vi "LSMcontroller_v59_PIzstage.vi"() -> ()   [LabVIEW 2015] (continued)
                        n916 = local write "64bit disabled"(TRUE ("64bit disabled")) -> ()
                      }
                      frame #9 {
                        n917 = call "2pparameters.vi"("command"="get") -> ("params out"=w3214:T11)  [unwired: 1 in]
                        n918 = Unbundle By Name(w3214) -> ("auto OD"=w3213:bool)
                        n919 = case shown="True" w3213 {
                          frame False {
                          }
                          frame True {
                            n920 = call "configuration.vi"("command"="get") -> ("config out"=w3217:T12)  [unwired: 2 in, 1 out]
                            n921 = call "2pparameters.vi"("command"="get") -> ("params out"=w3220:T11)  [unwired: 1 in]
                            n922 = Unbundle By Name(w3217) -> ("image OD"=w3215:u16)
                            n923 = Unbundle By Name(w3220) -> ("ODfilt"=w3216:u16)
                            n924 = call "filterwheelcontrol_nothorlabslib.vi"("Current OD filt"=w3215, "New ODfilt"=w3216) -> ()  [unwired: 1 in]
                          }
                        }
                        n925 = call "reset AO_DO_v3.vi"() -> ()  [unwired: 12 in]
                      }
                      frame #10 {
                        n926 = stacked-sequence {
                          tunnel: w3234 -> [w3237 _ _ _ _ _]
                          tunnel: w3233 -> [w3236 _ _ _ _ _]
                          tunnel: w3232 -> [w3235 _ _ _ _ _]
                          tunnel: w3231 -> [_ w3286 _ _ _ _]
                          tunnel: w3230 -> [_ w3285 w3340 w3437 _ _]
                          tunnel: w3229 -> [_ w3284 w3339 w3436 _ _]
                          tunnel: w3228 -> [_ _ w3338 _ _ _]
                          tunnel: w3227 -> [_ _ w3337 _ _ _]
                          tunnel: w3226 -> [_ _ _ w3435 _ _]
                          tunnel: w3225 -> [_ _ _ w3434 _ _]
                          tunnel: w3224 -> [_ _ w3335 _ _ _]
                          tunnel: w3223 -> [_ _ w3334 _ _ _]
                          tunnel: w3222 -> [_ _ _ w3432 _ _]
                          tunnel: w3221 -> [_ _ _ w3431 _ _]
                          frame #0 {
                            n927 = case shown="False" w3237 {
                              tunnel: w3236 -> [_ w3259]
                              tunnel: w3235 -> [_ w3258]
                              frame True {
                                n928 = stacked-sequence {
                                seq-local: [w3238 _ _] -> [_ w3250 w3255]
                                frame #0 {
                                n929 = call "configuration.vi"("command"="get") -> ("config out"=w3244:T12)  [unwired: 2 in, 1 out]
                                n930 = Unbundle By Name(w3244) -> ("Voltage to Xgalvo"=w3241:i32)
                                n931 = call "2pparameters.vi"("command"="get") -> ("params out"=w3242:T11)  [unwired: 1 in]
                                n932 = in-place {
                                in-place-border: w3241 -> [w3249]
                                in-place-border: [w3246] -> w3238
                                n933 = in-place-cluster #9(w3242) -> ("aAO"=w3248:u32[])
                                n934 = call "remove channel from active arrayv2.vi"("line array in"=w3248, "line to remove"=w3249) -> ("line array out"=w3247:u32[], "index"=w3246:i32)  [unwired: 1 out]
                                n935 = in-place-cluster #9("aAO"=w3247) -> (w3239:T11)
                                }
                                n936 = call "2pparameters.vi"("Params in"=w3239, "command"="set") -> ()  [unwired: 1 out]
                                }
                                frame #1 {
                                n937 = call "waveformparamsv2.vi"("command"="rem AO", "index"=w3250) -> ()  [unwired: 3 in, 3 out]
                                }
                                frame #2 {
                                n938 = call "waveformsAObuffer.vi"("command"="get") -> ("AO wf out"=w3256:waveform(dbl)[])  [unwired: 1 in]
                                n939 = Delete From Array(array=w3256, length=1, index=w3255) -> (array with subset deleted=w3252:waveform(dbl)[])  [unwired: 1 out]
                                n940 = call "waveformsAObuffer.vi"("AO wf in"=w3252, "command"="set") -> ()  [unwired: 1 out]
                                }
                                }
                              }
                              frame False {
                                n941 = stacked-sequence {
                                seq-local: [w3260 _ _] -> [_ w3268 w3279]
                                tunnel: w3259 -> [_ w3267 _]
                                tunnel: w3258 -> [_ _ w3278]
                                frame #0 {
                                n942 = call "configuration.vi"("command"="get") -> ("config out"=w3265:T12)  [unwired: 2 in, 1 out]
                                n943 = Unbundle By Name(w3265) -> ("Voltage to Xgalvo"=w3261:i32)
                                n944 = call "2pparameters.vi"("command"="get") -> ("params out"=w3264:T11)  [unwired: 1 in]
                                n945 = Unbundle By Name(w3264) -> ("aAO"=w3262:u32[])
                                n946 = Search 1D Array(1D array=w3262, element=w3261) -> (index of element=w3260:i32)  [unwired: 1 in]
                                }
                                frame #1 {
                                n947 = call "waveformparamsv2.vi"("command"="get") -> ("Params out"=w3271:T15)  [unwired: 4 in, 2 out]
                                n948 = in-place {
                                in-place-border: w3268 -> [w3275]
                                in-place-border: w3267 -> [w3274]
                                n949 = in-place-cluster #10(w3271) -> ("AO parameters"=w3276:T16)
                                n950 = in-place {
                                in-place-border: w3274 -> [w3277]
                                n951 = in-place-array #11(w3276, w3275) -> ()  [unwired: 1 out]
                                n952 = in-place-array #11(w3277) -> (w3273:T16)  [unwired: 1 out]
                                }
                                n953 = in-place-cluster #10("AO parameters"=w3273) -> (w3269:T15)
                                }
                                n954 = call "waveformparamsv2.vi"("command"="set", "Params in"=w3269) -> ()  [unwired: 3 in, 3 out]
                                }
                                frame #2 {
                                n955 = call "waveformsAObuffer.vi"("command"="get") -> ("AO wf out"=w3282:waveform(dbl)[])  [unwired: 1 in]
                                n956 = Replace Array Subset(array=w3282, new element=w3278, index=w3279) -> (w3280:waveform(dbl)[])
                                n957 = call "waveformsAObuffer.vi"("AO wf in"=w3280, "command"="set") -> ()  [unwired: 1 out]
                                }
                                }
                              }
                            }
                          }
                          frame #1 {
                            n958 = case shown="True" w3286 {
                              tunnel: w3285 -> [_ w3308]
                              tunnel: w3284 -> [_ w3307]
                              frame True {
                                n959 = stacked-sequence {
                                seq-local: [w3287 _ _] -> [_ w3299 w3304]
                                frame #0 {
                                n960 = call "configuration.vi"("command"="get") -> ("config out"=w3293:T12)  [unwired: 2 in, 1 out]
                                n961 = Unbundle By Name(w3293) -> ("Voltage to Ygalvo"=w3290:i32)
                                n962 = call "2pparameters.vi"("command"="get") -> ("params out"=w3291:T11)  [unwired: 1 in]
                                n963 = in-place {
                                in-place-border: w3290 -> [w3298]
                                in-place-border: [w3295] -> w3287
                                n964 = in-place-cluster #12(w3291) -> ("aAO"=w3297:u32[])
                                n965 = call "remove channel from active arrayv2.vi"("line array in"=w3297, "line to remove"=w3298) -> ("line array out"=w3296:u32[], "index"=w3295:i32)  [unwired: 1 out]
                                n966 = in-place-cluster #12("aAO"=w3296) -> (w3288:T11)
                                }
                                n967 = call "2pparameters.vi"("Params in"=w3288, "command"="set") -> ()  [unwired: 1 out]
                                }
                                frame #1 {
                                n968 = call "waveformparamsv2.vi"("command"="rem AO", "index"=w3299) -> ()  [unwired: 3 in, 3 out]
                                }
                                frame #2 {
                                n969 = call "waveformsAObuffer.vi"("command"="get") -> ("AO wf out"=w3305:waveform(dbl)[])  [unwired: 1 in]
                                n970 = Delete From Array(array=w3305, length=1, index=w3304) -> (array with subset deleted=w3301:waveform(dbl)[])  [unwired: 1 out]
                                n971 = call "waveformsAObuffer.vi"("AO wf in"=w3301, "command"="set") -> ()  [unwired: 1 out]
                                }
                                }
                              }
                              frame False {
                                n972 = stacked-sequence {
                                seq-local: [w3309 _ _] -> [_ w3317 w3328]
                                tunnel: w3308 -> [_ w3316 _]
                                tunnel: w3307 -> [_ _ w3327]
                                frame #0 {
                                n973 = call "configuration.vi"("command"="get") -> ("config out"=w3314:T12)  [unwired: 2 in, 1 out]
                                n974 = Unbundle By Name(w3314) -> ("Voltage to Ygalvo"=w3310:i32)
                                n975 = call "2pparameters.vi"("command"="get") -> ("params out"=w3313:T11)  [unwired: 1 in]
                                n976 = Unbundle By Name(w3313) -> ("aAO"=w3311:u32[])
                                n977 = Search 1D Array(1D array=w3311, element=w3310) -> (index of element=w3309:i32)  [unwired: 1 in]
                                }
                                frame #1 {
                                n978 = call "waveformparamsv2.vi"("command"="get") -> ("Params out"=w3320:T15)  [unwired: 4 in, 2 out]
                                n979 = in-place {
                                in-place-border: w3317 -> [w3324]
                                in-place-border: w3316 -> [w3323]
                                n980 = in-place-cluster #13(w3320) -> ("AO parameters"=w3325:T16)
                                n981 = in-place {
                                in-place-border: w3323 -> [w3326]
                                n982 = in-place-array #14(w3325, w3324) -> ()  [unwired: 1 out]
                                n983 = in-place-array #14(w3326) -> (w3322:T16)  [unwired: 1 out]
                                }
                                n984 = in-place-cluster #13("AO parameters"=w3322) -> (w3318:T15)
                                }
                                n985 = call "waveformparamsv2.vi"("command"="set", "Params in"=w3318) -> ()  [unwired: 3 in, 3 out]
                                }
                                frame #2 {
                                n986 = call "waveformsAObuffer.vi"("command"="get") -> ("AO wf out"=w3331:waveform(dbl)[])  [unwired: 1 in]
                                n987 = Replace Array Subset(array=w3331, new element=w3327, index=w3328) -> (w3329:waveform(dbl)[])
                                n988 = call "waveformsAObuffer.vi"("AO wf in"=w3329, "command"="set") -> ()  [unwired: 1 out]
                                }
                                }
                              }
                            }
                          }
                          frame #2 {
                            n989 = Build Array(w3335, w3334) -> (w3333:bool[])
                            n990 = Boolean Array To Number(Boolean array=w3333) -> (number=w3336:u32)
                            n991 = case shown="0" w3336 {
                              tunnel: w3340 -> [_ _ w3383]
                              tunnel: w3339 -> [_ _ w3382]
                              tunnel: w3338 -> [_ w3362 w3380]
                              tunnel: w3337 -> [_ w3361 w3381]
                              frame 1, Default {
                                n992 = stacked-sequence {
                                seq-local: [w3341 _ _] -> [_ w3353 w3358]
                                frame #0 {
                                n993 = call "configuration.vi"("command"="get") -> ("config out"=w3347:T12)  [unwired: 2 in, 1 out]
                                n994 = Unbundle By Name(w3347) -> ("2P shutter"=w3344:i32)
                                n995 = call "2pparameters.vi"("command"="get") -> ("params out"=w3345:T11)  [unwired: 1 in]
                                n996 = in-place {
                                in-place-border: w3344 -> [w3352]
                                in-place-border: [w3349] -> w3341
                                n997 = in-place-cluster #15(w3345) -> ("aDO"=w3351:u32[])
                                n998 = call "remove channel from active arrayv2.vi"("line array in"=w3351, "line to remove"=w3352) -> ("line array out"=w3350:u32[], "index"=w3349:i32)  [unwired: 1 out]
                                n999 = in-place-cluster #15("aDO"=w3350) -> (w3342:T11)
                                }
                                n1000 = call "2pparameters.vi"("Params in"=w3342, "command"="set") -> ()  [unwired: 1 out]
                                }
                                frame #1 {
                                n1001 = call "waveformparamsv2.vi"("command"="rem DO", "index"=w3353) -> ()  [unwired: 3 in, 3 out]
                                }
                                frame #2 {
                                n1002 = call "waveformsDObuffer.vi"("command"="get") -> ("DO wf out"=w3359:digitalwaveform[])  [unwired: 1 in]
                                n1003 = Delete From Array(array=w3359, length=1, index=w3358) -> (array with subset deleted=w3355:digitalwaveform[])  [unwired: 1 out]
                                n1004 = call "waveformsDObuffer.vi"("DO wf in"=w3355, "command"="set") -> ()  [unwired: 1 out]
                                }
                                }
                              }
                              frame 2 {
                                n1005 = stacked-sequence {
                                tunnel: w3362 -> [_ w3373 _]
                                tunnel: w3361 -> [_ _ w3377]
                                frame #0 {
                                n1006 = call "configuration.vi"("command"="get") -> ("config out"=w3364:T12)  [unwired: 2 in, 1 out]
                                n1007 = call "2pparameters.vi"("command"="get") -> ("params out"=w3368:T11)  [unwired: 1 in]
                                n1008 = Unbundle By Name(w3364) -> ("2P shutter"=w3363:i32)
                                n1009 = in-place {
                                in-place-border: w3363 -> [w3372]
                                n1010 = in-place-cluster #16(w3368) -> ("aDO"=w3371:u32[])
                                n1011 = call "add channel to active arrayv2.vi"("line array in"=w3371, "line to add"=w3372) -> ("line array out"=w3370:u32[])  [unwired: 2 out]
                                n1012 = in-place-cluster #16("aDO"=w3370) -> (w3366:T11)
                                }
                                n1013 = call "2pparameters.vi"("Params in"=w3366, "command"="set") -> ()  [unwired: 1 out]
                                }
                                frame #1 {
                                n1014 = call "waveformparamsv2.vi"("command"="add DO", "add DO"=w3373) -> ()  [unwired: 3 in, 3 out]
                                }
                                frame #2 {
                                n1015 = call "waveformsDObuffer.vi"("command"="get") -> ("DO wf out"=w3378:digitalwaveform[])  [unwired: 1 in]
                                n1016 = Build Array (concatenate)(w3378, w3377) -> (w3376:digitalwaveform[])
                                n1017 = call "waveformsDObuffer.vi"("DO wf in"=w3376, "command"="set") -> ()  [unwired: 1 out]
                                }
                                }
                              }
                              frame 0 {
                                n1018 = stacked-sequence {
                                seq-local: [w3384 _ _] -> [_ w3392 w3414]
                                tunnel: w3383 -> [_ _ _]
                                tunnel: w3382 -> [_ _ _]
                                tunnel: w3381 -> [_ _ w3413]
                                tunnel: w3380 -> [_ w3391 _]
                                frame #0 {
                                n1019 = call "configuration.vi"("command"="get") -> ("config out"=w3389:T12)  [unwired: 2 in, 1 out]
                                n1020 = call "2pparameters.vi"("command"="get") -> ("params out"=w3388:T11)  [unwired: 1 in]
                                n1021 = Unbundle By Name(w3389) -> ("2P shutter"=w3385:i32)
                                n1022 = Unbundle By Name(w3388) -> ("aDO"=w3386:u32[])
                                n1023 = Search 1D Array(1D array=w3386, element=w3385) -> (index of element=w3384:i32)  [unwired: 1 in]
                                }
                                frame #1 {
                                n1024 = call "2pparameters.vi"("command"="get") -> ("params out"=w3395:T11)  [unwired: 1 in]
                                n1025 = Unbundle By Name(w3395) -> ("wavdet"=w3393:bool, "autoshutter"=w3394:bool)
                                n1026 = case shown="True" w3394 {
                                tunnel: w3392 -> [_ w3399]
                                tunnel: w3393 -> [_ w3398]
                                tunnel: w3391 -> [_ w3397]
                                frame False {
                                }
                                frame True {
                                n1027 = case shown="False" w3398 {
                                tunnel: w3399 -> [w3403 _]
                                tunnel: w3397 -> [w3401 _]
                                frame False {
                                n1028 = Index Array(array=w3401, index=0) -> (element=w3400:T19)
                                n1029 = call "waveformparamsv2.vi"("command"="get") -> ("Params out"=w3406:T15)  [unwired: 4 in, 2 out]
                                n1030 = in-place {
                                in-place-border: w3403 -> [w3410]
                                in-place-border: w3400 -> [w3408]
                                n1031 = in-place-cluster #17(w3406) -> ("DO parameters"=w3411:T18)
                                n1032 = in-place {
                                in-place-border: w3408 -> [w3412]
                                n1033 = in-place-array #18(w3411, w3410) -> ()  [unwired: 1 out]
                                n1034 = in-place-array #18(w3412) -> (w3409:T18)  [unwired: 1 out]
                                }
                                n1035 = in-place-cluster #17("DO parameters"=w3409) -> (w3404:T15)
                                }
                                n1036 = call "waveformparamsv2.vi"("command"="set", "Params in"=w3404) -> ()  [unwired: 3 in, 3 out]
                                }
                                frame True {
                                }
                                }
                                }
                                }
                                }
                                frame #2 {
                                n1037 = call "2pparameters.vi"("command"="get") -> ("params out"=w3417:T11)  [unwired: 1 in]
                                n1038 = Unbundle By Name(w3417) -> ("wavdet"=w3415:bool, "autoshutter"=w3416:bool)
                                n1039 = case shown="True" w3416 {
                                tunnel: w3414 -> [_ w3421]
                                tunnel: w3415 -> [_ w3420]
                                tunnel: w3413 -> [_ w3419]
                                frame False {
                                }
                                frame True {
                                n1040 = case shown="False" w3420 {
                                tunnel: w3421 -> [w3425 _]
                                tunnel: w3419 -> [w3424 _]
                                frame False {
                                n1041 = Index Array(array=w3424, index=0) -> (element=w3422:digitalwaveform)
                                n1042 = call "waveformsDObuffer.vi"("command"="get") -> ("DO wf out"=w3427:digitalwaveform[])  [unwired: 1 in]
                                n1043 = Replace Array Subset(array=w3427, new element=w3422, index=w3425) -> (w3429:digitalwaveform[])
                                n1044 = call "waveformsDObuffer.vi"("DO wf in"=w3429, "command"="set") -> ()  [unwired: 1 out]
                                }
                                frame True {
                                }
                                }
                                }
                                }
                                }
                                }
                              }
                            }
                          }
                          frame #3 {
                            n1045 = Build Array(w3432, w3431) -> (w3433:bool[])
                            n1046 = Boolean Array To Number(Boolean array=w3433) -> (number=w3430:u32)
                            n1047 = case shown="0" w3430 {
                              tunnel: w3437 -> [_ _ w3480]
                              tunnel: w3436 -> [_ _ w3479]
                              tunnel: w3435 -> [_ w3459 w3477]
                              tunnel: w3434 -> [_ w3458 w3478]
                              frame 1, Default {
                                n1048 = stacked-sequence {
                                seq-local: [w3438 _ _] -> [_ w3450 w3455]
                                frame #0 {
                                n1049 = call "configuration.vi"("command"="get") -> ("config out"=w3444:T12)  [unwired: 2 in, 1 out]
                                n1050 = Unbundle By Name(w3444) -> ("LT timestamp"=w3441:u32)
                                n1051 = call "2pparameters.vi"("command"="get") -> ("params out"=w3442:T11)  [unwired: 1 in]
                                n1052 = in-place {
                                in-place-border: w3441 -> [w3449]
                                in-place-border: [w3446] -> w3438
                                n1053 = in-place-cluster #19(w3442) -> ("aDO"=w3448:u32[])
                                n1054 = call "remove channel from active arrayv2.vi"("line array in"=w3448, "line to remove"=w3449) -> ("line array out"=w3447:u32[], "index"=w3446:i32)  [unwired: 1 out]
                                n1055 = in-place-cluster #19("aDO"=w3447) -> (w3439:T11)
                                }
                                n1056 = call "2pparameters.vi"("Params in"=w3439, "command"="set") -> ()  [unwired: 1 out]
                                }
                                frame #1 {
                                n1057 = call "waveformparamsv2.vi"("command"="rem DO", "index"=w3450) -> ()  [unwired: 3 in, 3 out]
                                }
                                frame #2 {
                                n1058 = call "waveformsDObuffer.vi"("command"="get") -> ("DO wf out"=w3456:digitalwaveform[])  [unwired: 1 in]
                                n1059 = Delete From Array(array=w3456, length=1, index=w3455) -> (array with subset deleted=w3452:digitalwaveform[])  [unwired: 1 out]
                                n1060 = call "waveformsDObuffer.vi"("DO wf in"=w3452, "command"="set") -> ()  [unwired: 1 out]
                                }
                                }
                              }
                              frame 2 {
                                n1061 = stacked-sequence {
                                tunnel: w3459 -> [_ _ w3472]
                                tunnel: w3458 -> [_ w3470 _]
                                frame #0 {
                                n1062 = call "configuration.vi"("command"="get") -> ("config out"=w3461:T12)  [unwired: 2 in, 1 out]
                                n1063 = Unbundle By Name(w3461) -> ("LT timestamp"=w3460:u32)
                                n1064 = call "2pparameters.vi"("command"="get") -> ("params out"=w3465:T11)  [unwired: 1 in]
                                n1065 = in-place {
                                in-place-border: w3460 -> [w3469]
                                n1066 = in-place-cluster #20(w3465) -> ("aDO"=w3468:u32[])
                                n1067 = call "add channel to active arrayv2.vi"("line array in"=w3468, "line to add"=w3469) -> ("line array out"=w3467:u32[])  [unwired: 2 out]
                                n1068 = in-place-cluster #20("aDO"=w3467) -> (w3463:T11)
                                }
                                n1069 = call "2pparameters.vi"("Params in"=w3463, "command"="set") -> ()  [unwired: 1 out]
                                }
                                frame #1 {
                                n1070 = call "waveformparamsv2.vi"("command"="add DO", "add DO"=w3470) -> ()  [unwired: 3 in, 3 out]
                                }
                                frame #2 {
                                n1071 = call "waveformsDObuffer.vi"("command"="get") -> ("DO wf out"=w3475:digitalwaveform[])  [unwired: 1 in]
                                n1072 = Build Array (concatenate)(w3475, w3472) -> (w3474:digitalwaveform[])
                                n1073 = call "waveformsDObuffer.vi"("DO wf in"=w3474, "command"="set") -> ()  [unwired: 1 out]
                                }
                                }
                              }
                              frame 0 {
                                n1074 = stacked-sequence {
                                seq-local: [w3481 _ _] -> [_ w3491 w3508]
                                tunnel: w3480 -> [_ _ _]
                                tunnel: w3479 -> [_ _ _]
                                tunnel: w3478 -> [_ w3488 _]
                                tunnel: w3477 -> [_ _ w3507]
                                frame #0 {
                                n1075 = call "configuration.vi"("command"="get") -> ("config out"=w3486:T12)  [unwired: 2 in, 1 out]
                                n1076 = Unbundle By Name(w3486) -> ("LT timestamp"=w3482:u32)
                                n1077 = call "2pparameters.vi"("command"="get") -> ("params out"=w3485:T11)  [unwired: 1 in]
                                n1078 = Unbundle By Name(w3485) -> ("aDO"=w3483:u32[])
                                n1079 = Search 1D Array(1D array=w3483, element=w3482) -> (index of element=w3481:i32)  [unwired: 1 in]
                                }
                                frame #1 {
                                n1080 = local read "Measurement"() -> (w3490:T4)
                                n1081 = To Unsigned Long Integer(number=w3490) -> (unsigned 32bit integer=w3489:u32)
                                n1082 = case shown="5..7" w3489 {
                                tunnel: w3491 -> [_ w3495]
                                tunnel: w3488 -> [_ w3492]
                                frame 0..4, Default {
                                }
                                frame 5..7 {
                                n1083 = Index Array(array=w3492, index=0) -> (element=w3493:T19)
                                n1084 = call "waveformparamsv2.vi"("command"="get") -> ("Params out"=w3498:T15)  [unwired: 4 in, 2 out]
                                n1085 = in-place {
                                in-place-border: w3495 -> [w3502]
                                in-place-border: w3493 -> [w3500]
                                n1086 = in-place-cluster #21(w3498) -> ("DO parameters"=w3503:T18)
                                n1087 = in-place {
                                in-place-border: w3500 -> [w3504]
                                n1088 = in-place-array #22(w3503, w3502) -> ()  [unwired: 1 out]
                                n1089 = in-place-array #22(w3504) -> (w3501:T18)  [unwired: 1 out]
                                }
                                n1090 = in-place-cluster #21("DO parameters"=w3501) -> (w3496:T15)
                                }
                                n1091 = call "waveformparamsv2.vi"("command"="set", "Params in"=w3496) -> ()  [unwired: 3 in, 3 out]
                                }
                                }
                                }
                                frame #2 {
                                n1092 = local read "Measurement"() -> (w3506:T4)
                                n1093 = To Unsigned Long Integer(number=w3506) -> (unsigned 32bit integer=w3505:u32)
                                n1094 = case shown="5..7" w3505 {
                                tunnel: w3508 -> [_ w3512]
                                tunnel: w3507 -> [_ w3510]
                                frame 0..4, Default {
                                }
                                frame 5..7 {
                                n1095 = Index Array(array=w3510, index=0) -> (element=w3509:digitalwaveform)
                                n1096 = call "waveformsDObuffer.vi"("command"="get") -> ("DO wf out"=w3514:digitalwaveform[])  [unwired: 1 in]
                                n1097 = Replace Array Subset(array=w3514, new element=w3509, index=w3512) -> (w3516:digitalwaveform[])
                                n1098 = call "waveformsDObuffer.vi"("DO wf in"=w3516, "command"="set") -> ()  [unwired: 1 out]
                                }
                                }
                                }
                                }
                              }
                            }
                          }
                          frame #4 {
                            n1099 = call "Used AO lines.vi"() -> ("used AO names"=w3519:string[], "used AO lines"=w3517:tag[])  [unwired: 2 in]
                            n1100 = control-ref of="Analog Lines Plot"() -> (w3518:refnum<vi>)
                            n1101 = control-ref of="Digital Lines Plot"() -> (w3520:refnum<vi>)
                            n1102 = call "Used DO lines.vi"() -> ("used DO names"=w3521:string[], "used DO lines"=w3522:tag[])  [unwired: 2 in]
                            n1103 = local write "Analog Used Lines"(w3517) -> ()
                            n1104 = local write "Analog Used Names"(w3519) -> ()
                            n1105 = local write "Digital Used Lines"(w3522) -> ()
                            n1106 = local write "Digital Used Names"(w3521) -> ()
                            n1107 = call "prepDOWaveplot.vi"("DigitalGraph in"=w3520, "used DO names"=w3521) -> ()  [unwired: 1 in]
                            n1108 = call "prepAOWaveplot.vi"("WaveformGraph in"=w3518, "Analog Used Names"=w3519) -> ()  [unwired: 1 in]
                          }
                          frame #5 {
                            n1109 = local read "Meastab"() -> (w3537:enum32{"X-Y Image", "Linescan", "Timetrace"})
                            n1110 = property on="refwf" class="Ring (strict)"() -> ("RingText.Text"=w3534:string)  [unwired: 2 in, 2 out]
                            n1111 = case shown="\"Timetrace\"" w3537 {
                              tunnel: [w3539 w3540] -> w3538
                              frame "X-Y Image", Default {
                                n1112 = local read "Sampling rate"() -> (w3539:dbl)
                              }
                              frame "Timetrace" {
                                n1113 = local read "srateAODOtt"() -> (w3540:dbl)
                              }
                            }
                            n1114 = call "waveformsAObuffer.vi"("command"="get") -> ("AO wf out"=w3525:waveform(dbl)[])  [unwired: 1 in]
                            n1115 = local read "wavdet"() -> (w3535:bool)
                            n1116 = call "waveformsDObuffer.vi"("command"="get") -> ("DO wf out"=w3529:digitalwaveform[])  [unwired: 1 in]
                            n1117 = call "correctwaveformsizetemp.vi"("new sampling frequency (Hz)"=w3538, "start"=FALSE, "reference waveforms to"=w3534, "Analog waveforms in"=w3525, "stop"=TRUE, "Digital waveforms in"=w3529) -> ("analog wf out"=w3531:waveform(dbl)[], "Digital wf out"=w3533:digitalwaveform[], "measpoints"=w3536:i32)
                            n1118 = local write "Analog Lines Plot"(w3531) -> ()
                            n1119 = call "GetNumCamFramesv2.vi"("Digital Waveform Graph"=w3533) -> ("Numeric"=w3532:i32)  [unwired: 10 in]
                            n1120 = local write "Digital Lines Plot"(w3533) -> ()
                            n1121 = call "waveformsDObuffer.vi"("DO wf in"=w3533, "command"="set") -> ()  [unwired: 1 out]
                            n1122 = call "waveformsAObuffer.vi"("AO wf in"=w3531, "command"="set") -> ()  [unwired: 1 out]
                            n1123 = local write "Total Camera Frames"(w3532) -> ()
                            n1124 = case shown="True" w3535 {
                              tunnel: w3536 -> [_ w3541]
                              frame False {
                              }
                              frame True {
                                n1125 = local write "# of frames"(w3541) -> ()
                              }
                            }
                          }
                        }
                        n1126 = call "stoperaseCI.vi"() -> ()  [unwired: 12 in]
                        n1127 = call "stoperaseDO_img.vi"() -> ()  [unwired: 12 in]
                        n1128 = call "stoperaseAO_img.vi"() -> ()  [unwired: 12 in]
                        n1129 = call "stoperaseAI_img.vi"() -> ()  [unwired: 12 in]
                      }
                      frame #11 {
                        w3549 = FALSE ("Value (Signaling)")
                        n1130 = local read "save\ndata"() -> (w3542:bool)
                        n1131 = local read "save\ndata"() -> (w3543:bool)
                        n1132 = property on="Stop" class="Bool (strict)"("Visible"=FALSE, "DisabledEnum"=T7."Disabled" ("Disabled")) -> ()  [unwired: 2 in, 2 out]
                        n1133 = case shown="True" w3542 {
                          frame False {
                          }
                          frame True {
                            n1134 = call "closetiffs.vi"() -> ()  [unwired: 12 in]
                          }
                        }
                        n1135 = case shown="True" w3543 {
                          tunnel: w3544 -> [_ w3550]
                          frame False {
                          }
                          frame True {
                            n1136 = local read "filename prefix"() -> (w3552:string)
                            n1137 = local read "data dir"() -> (w3551:path)
                            n1138 = call "savetimestamps.vi"("timestamp"=w3550, "filename prefix in"=w3552, "data dir in"=w3551) -> ()  [unwired: 1 in]
                            n1139 = call "saveparams.vi"("filename prefix in"=w3552, "data dir in"=w3551) -> ()  [unwired: 2 in]
                          }
                        }
                        n1140 = property on="Start" class="Bool (strict)"("Visible"=TRUE, "DisabledEnum"=T7."Enabled" ("Disabled")) -> ()  [unwired: 2 in, 2 out]
                        n1141 = property on="Start" class="Bool (strict)"("Val(Sgnl)"=w3549) -> ()  [unwired: 2 in, 2 out]
                        n1142 = property on="Stop" class="Bool (strict)"("Val(Sgnl)"=w3549) -> ()  [unwired: 2 in, 2 out]
                      }
                      frame #12 {
                        w3556 = T22 2 items=["no dialog", "OK message", "continue or stop message", "OK message + warnings", "continue/stop + warnings"] ("type of dialog (OK msg:1)")
                        n1143 = call "displayerrors.vi"() -> ("error IO"=w3555:errorcluster)
                        n1144 = call <vilib>:"General Error Handler.vi"("type of dialog (OK msg:1)"=w3556, "error in (no error)"=w3555) -> ("error out"=w3554:errorcluster)  [unwired: 9 in, 4 out]
                        n1145 = call <vilib>:"Clear Errors.vi"("error in (no error)"=w3554) -> ("error out"=w3553:errorcluster)  [unwired: 5 in, 1 out]
                        n1146 = call "seterrors.vi"("error IO"=w3553) -> ()
                      }
                    }
                  }
                  frame "X-Y-Z-t movie" {
                    n1147 = call "2pparameters.vi"("command"="get") -> ("params out"=w3559:T11)  [unwired: 1 in]
                    n1148 = Bundle By Name(cluster=w3559, "type"="X-Y-Z-t movie") -> (w3557:T11)
                    n1149 = call "2pparameters.vi"("Params in"=w3557, "command"="set") -> ()  [unwired: 1 out]
                  }
                  frame "linescan" {
                    n1150 = call "2pparameters.vi"("command"="get") -> ("params out"=w3564:T11)  [unwired: 1 in]
                    n1151 = Bundle By Name(cluster=w3564, "type"="linescan") -> (w3566:T11)
                    n1152 = call "2pparameters.vi"("Params in"=w3566, "command"="set") -> ()  [unwired: 1 out]
                  }
                  frame "Timetrace", "Lifetime (contour)" {
                    n1153 = local read "ttt"() -> (w3567:T3)
                    n1154 = case shown="\"Resonant Ellipse\", \"freeform contour\"" w3567 {
                      frame "Point", Default {
                        n1155 = stacked-sequence {
                          seq-local: [w3568 _ _ _ _ _ _ _ _] -> [_ _ w3701 _ _ _ _ _ w3759]
                          frame #0 {
                            n1156 = Get Date/Time In Seconds() -> (seconds since 1Jan1904=w3569:timestamp)
                            n1157 = call "createdatafolder.vi"("timestamp in"=w3569) -> ("current data path"=w3570:path, "timestamp out"=w3568:timestamp)
                            n1158 = stacked-sequence {
                              frame #0 {
                                n1159 = call "2pparameters.vi"("command"="get") -> ("params out"=w3585:T11)  [unwired: 1 in]
                                n1160 = Bundle By Name(cluster=w3585, "type"="Timetrace") -> (w3583:T11)
                                n1161 = call "2pparameters.vi"("command"="get") -> ("params out"=w3574:T11)  [unwired: 1 in]
                                n1162 = local write "graphtab"(T5."timetrace" ("graphtab")) -> ()
                                n1163 = Unbundle By Name(w3574) -> ("Vx-min Img"=w3576:dbl, "VX-max Img"=w3575:dbl, "Vy-min Img"=w3578:dbl, "Vy-max Img"=w3577:dbl, "Angle Img"=w3579:dbl)
                                n1164 = property on="Stop" class="Bool (strict)"("Visible"=TRUE, "DisabledEnum"=T7."Enabled" ("Disabled")) -> ()  [unwired: 2 in, 2 out]
                                n1165 = property on="Start" class="Bool (strict)"("Visible"=FALSE, "DisabledEnum"=T7."Disabled and Grayed Out" ("Disabled")) -> ()  [unwired: 2 in, 2 out]
                                n1166 = local read "Vy-ref"() -> (w3581:dbl)
                                n1167 = local read "Vx-ref"() -> (w3580:dbl)
                                n1168 = call "2pparameters.vi"("Params in"=w3583, "command"="set") -> ()  [unwired: 1 out]
                                n1169 = script code="Xic=(ximax+ximin)./2;\nYic=(yimax+yimin)./2;\nx=x-Xic;\ny=y-Yic;\nxout=x.*cos(pi/180.*phi)+y.*sin(pi./180.*phi)+Xic;\nyout=-x.*sin(pi./180.*phi)+y.*cos(pi./180.*phi)+Yic;"("ximax"=w3575, "ximin"=w3576, "yimax"=w3577, "yimin"=w3578, "phi"=w3579, "x"=w3580, "y"=w3581) -> ("xout"=w3572:dbl, "yout"=w3571:dbl)  [unwired: 1 in, 1 out]
                                n1170 = call "setposition.vi"("Vy"=w3571, "Vx"=w3572) -> ()  [unwired: 1 in]
                              }
                              frame #1 {
                                n1171 = call "2pparameters.vi"("command"="get") -> ("params out"=w3594:T11)  [unwired: 1 in]
                                n1172 = Unbundle By Name(w3594) -> ("autoshutter"=w3595:bool, "auto OD"=w3592:bool)
                                n1173 = case shown="True" w3592 {
                                frame False {
                                }
                                frame True {
                                n1174 = call "configuration.vi"("command"="get") -> ("config out"=w3598:T12)  [unwired: 2 in, 1 out]
                                n1175 = Unbundle By Name(w3598) -> ("point OD"=w3599:u16)
                                n1176 = local read "ODfilt"() -> (w3596:u16)
                                n1177 = call "filterwheelcontrol_nothorlabslib.vi"("Current OD filt"=w3596, "New ODfilt"=w3599) -> ()  [unwired: 1 in]
                                }
                                }
                                n1178 = case shown="True" w3595 {
                                frame False {
                                }
                                frame True {
                                n1179 = call "shuttercontrol.vi"("command"="close") -> ()  [unwired: 1 in, 1 out]
                                }
                                }
                              }
                              frame #2 {
                                n1180 = local read "refreshtime"() -> (w3604:dbl)
                                n1181 = local read "wavdet"() -> (w3620:bool)
                                n1182 = local read "finite samples"() -> (w3619:bool)
                                n1183 = local read "srateAODOtt"() -> (w3605:dbl)
                                n1184 = local read "srateAODOtt"() -> (w3621:dbl)
                                n1185 = local read "srateAODOtt"() -> (w3606:dbl)
                                n1186 = Multiply(x=w3605, y=w3604) -> (x*y=w3615:dbl)
                                n1187 = local read "# of frames"() -> (w3614:i32)
                                n1188 = Reciprocal(x=w3604) -> (1/x=w3603:dbl)
                                n1189 = To Long Integer(number=w3615) -> (32bit integer=w3613:i32)
                                n1190 = Quotient & Remainder(x=w3614, y=w3613) -> (x-y*floor(x/y)=w3610:i32, floor(x/y)=w3607:i32)
                                n1191 = local read "AI channels"() -> (w3602:i32[])
                                n1192 = local read "CI channels"() -> (w3601:i32[])
                                n1193 = Equal To 0?(x=w3610) -> (x = 0?=w3609:bool)
                                n1194 = Increment(x=w3607) -> (x+1=w3608:i32)
                                n1195 = local read "continuous"() -> (w3618:bool)
                                n1196 = local read "Vx-ref"() -> (w3612:dbl)
                                n1197 = local read "Vy-ref"() -> (w3617:dbl)
                                n1198 = Select(t=w3607, s=w3609, f=w3608) -> (s? t:f=w3611:i32)
                                n1199 = local read "avpp"() -> (w3616:i32)
                                n1200 = call "2pparameters.vi"("command"="get") -> ("params out"=w3624:T11)  [unwired: 1 in]
                                n1201 = Bundle By Name(cluster=w3624, "measpoints"=w3614, "tt_cycles"=w3611, "refreshbuffer"=w3613, "refreshrate"=w3603, "Vx-ref"=w3612, "Vy-ref"=w3617, "srate"=w3621, "finite"=w3619, "cont"=w3618, "wavdet"=w3620, "avpp"=w3616, "srateAODO"=w3606, "aAI"=w3602, "aCI"=w3601) -> (w3622:T11)
                                n1202 = call "2pparameters.vi"("Params in"=w3622, "command"="set") -> ()  [unwired: 1 out]
                              }
                              frame #3 {
                                n1203 = local read "Vholding (mV)"() -> (w3627:sgl)
                                n1204 = local read "Current Clamp"() -> (w3633:bool)
                                n1205 = local read "Voltage Clamp"() -> (w3632:bool)
                                n1206 = local read "OCgain"() -> (w3628:sgl)
                                n1207 = local read "CC_ICgain"() -> (w3631:dbl)
                                n1208 = local read "holdon"() -> (w3626:bool)
                                n1209 = call "patchparameters.vi"("command"="get") -> ("Params out"=w3635:T14)  [unwired: 1 in]
                                n1210 = Bundle By Name(cluster=w3635, "VC"=w3632, "CC"=w3633, "CC_icg (pA/mv)"=w3631, "VC_icg (mV/mV)"=10.0, "OCG (mV/pA)"=w3628, "OVG (mV/mV)"=0.1, "Vhold (mV)"=w3627, "holdon"=w3626) -> (w3634:T14)
                                n1211 = call "patchparameters.vi"("Params in"=w3634, "command"="set") -> ()  [unwired: 1 out]
                              }
                              frame #4 {
                                n1212 = local read "wavdet"() -> (w3638:bool)
                                n1213 = case shown="True" w3638 {
                                frame False {
                                }
                                frame True {
                                n1214 = stacked-sequence {
                                frame #0 {
                                n1215 = disable-structure shown="Disabled" {
                                frame Disabled {
                                w3650 = 10178 items=["Finite Samples"=10178, "Continuous Samples"=10123, "Hardware Timed Single Point"=12522] ("sample mode")
                                n1216 = call "patchparameters.vi"("command"="get") -> ("Params out"=w3643:T14)  [unwired: 1 in]
                                n1217 = Unbundle By Name(w3643) -> ("CC"=w3644:bool)
                                n1218 = case shown="True" w3644 {
                                tunnel: [w3661 w3664] -> w3641
                                frame False {
                                n1219 = call "patchparameters.vi"("command"="get") -> ("Params out"=w3662:T14)  [unwired: 1 in]
                                n1220 = Unbundle By Name(w3662) -> ("VC_icg (mV/mV)"=w3661:sgl)
                                }
                                frame True {
                                n1221 = call "patchparameters.vi"("command"="get") -> ("Params out"=w3665:T14)  [unwired: 1 in]
                                n1222 = Unbundle By Name(w3665) -> ("CC_icg (pA/mv)"=w3664:sgl)
                                }
                                }
                                n1223 = local read "refreshtime"() -> (w3640:dbl)
                                n1224 = local read "srateAODOtt"() -> (w3651:dbl)
                                n1225 = local read item#-1() -> (w3654)
                                n1226 = local read item#-1() -> (w3660)
                                n1227 = local read item#-1() -> (w3653)
                                n1228 = local read item#-1() -> (w3658)
                                n1229 = local read item#-1() -> (w3652)
                                n1230 = local read item#-1() -> (w3659)
                                n1231 = local read item#-1() -> (w3657)
                                n1232 = local read item#-1() -> (w3655)
                                n1233 = local read item#-1() -> (w3656)
                                n1234 = Reciprocal(x=w3640) -> (1/x=w3639:dbl)
                                n1235 = call "waveformparamsv2.vi"("command"="get") -> ("Params out"=w3647:T23)  [unwired: 1 in]
                                n1236 = Bundle By Name(cluster=w3647, "AO parameters"=w3652, "DO parameters"=w3653, "Duty cycle sq(%)"=w3654, "Voltage freq. sq(Hz)"=w3655, "# cycles sq"=w3656, "meastype"=T9."Manual", "sample rate"=w3651, "amp"=w3641, "sample mode"=w3650, "Min Voltage tri (mV)"=w3657, "Max voltage tri (mV)"=w3658, "Voltage freq. tri(Hz)"=w3659, "# cycles tri"=w3660, "refreshrate"=w3639) -> (w3648:T23)
                                n1237 = call "waveformparamsv2.vi"("Params in"=w3648, "command"="set") -> ()  [unwired: 1 out]
                                }
                                frame Enabled {
                                }
                                }
                                }
                                frame #1 {
                                n1238 = disable-structure shown="Disabled" {
                                frame Disabled {
                                n1239 = call "2pparameters.vi"("command"="set") -> ("params out"=w3669:T11)  [unwired: 1 in]
                                n1240 = local read item#-1() -> (w3676)
                                n1241 = local read item#-1() -> (w3675)
                                n1242 = local read item#-1() -> (w3677)
                                n1243 = Unbundle By Name(w3669) -> ("aAO"=w3668:u32[], "aDO"=w3667:u32[])
                                n1244 = call "waveformparamsv2.vi"("command"="get") -> ("Params out"=w3673:T23)  [unwired: 1 in]
                                n1245 = Bundle By Name(cluster=w3673, "lAO"=w3668, "lDO"=w3667, "Voltage step"=w3675, "Voltage triangle"=w3677, "file"=w3676) -> (w3674:T23)
                                n1246 = call "waveformparamsv2.vi"("Params in"=w3674, "command"="set") -> ()  [unwired: 1 out]
                                }
                                frame Enabled {
                                }
                                }
                                }
                                frame #2 {
                                n1247 = disable-structure shown="Disabled" {
                                frame Disabled {
                                n1248 = local read item#-1() -> (w3679)
                                n1249 = call "load waveforms.vi"("waveform"=w3679) -> ("# of points"=w3678:i32)
                                n1250 = local write "# of frames"(w3678) -> ()
                                }
                                frame Enabled {
                                }
                                }
                                }
                                }
                                }
                                }
                              }
                              frame #5 {
                                n1251 = call "2pparameters.vi"("command"="get") -> ("params out"=w3690:T11)  [unwired: 1 in]
                                n1252 = Unbundle By Name(w3690) -> ("refreshbuffer"=w3688:i32, "srate"=w3689:sgl)
                                n1253 = local read "wavdet"() -> (w3682:bool)
                                n1254 = case shown="True" w3682 {
                                tunnel: [w3697 w3698] -> w3681
                                frame False {
                                w3697 = 10123 items=["Finite Samples"=10178, "Continuous Samples"=10123, "Hardware Timed Single Point"=12522] ("sample mode")
                                }
                                frame True {
                                w3698 = 10123 items=["Finite Samples"=10178, "Continuous Samples"=10123, "Hardware Timed Single Point"=12522] ("sample mode")
                                }
                                }
                                n1255 = To Double Precision Float(number=w3689) -> (double precision float=w3692:dbl)
                                n1256 = To Double Precision Float(number=w3688) -> (double precision float=w3683:dbl)
                                n1257 = Divide(x=w3683, y=w3692) -> (x/y=w3696:dbl)
                                n1258 = Multiply(x=w3696, y=2.0) -> (x*y=w3693:dbl)
                                n1259 = Max & Min(x=w3693, y=10.0) -> (max(x,y)=w3684:dbl)  [unwired: 1 out]
                                n1260 = call "2pparameters.vi"("command"="get") -> ("params out"=w3687:T11)  [unwired: 1 in]
                                n1261 = Bundle By Name(cluster=w3687, "timeout"=w3684, "sample mode"=w3681) -> (w3685:T11)
                                n1262 = call "2pparameters.vi"("Params in"=w3685, "command"="set") -> ()  [unwired: 1 out]
                              }
                            }
                            n1263 = local write "data dir"(w3570) -> ()
                          }
                          frame #1 {
                            # "determine size of AI buffer still!!!"
                            # "counter needs a clock. rather than setting up a separate clock line\n (i have no more counters) I opt to always record an AI channel;\nin imaging i don't do this because the scanner provides a clock and the\nspeed needed to record at appreciable framerates makes it useful to limit the number of channels.\nin timetrace, the samplerate is unlikely to ever go over >10Ks/s so it matters less."
                            # "shutter line"
                            # "to patch and\nlaser (eventual aotf)"
                            n1264 = call "prepAO_tt_v2.vi"() -> ("Terminal Name with Device Prefix"=w3699:tag)  [unwired: 2 in]
                            n1265 = call "prepDO_tt.vi"() -> ()  [unwired: 2 in]
                            n1266 = call "prepAI_ttv2.vi"("triggersource"=w3699) -> ()  [unwired: 1 in, 1 out]
                            n1267 = call "prepCI_tt.vi"() -> ()  [unwired: 2 in]
                          }
                          frame #2 {
                            n1268 = local read "save\ndata"() -> (w3700:bool)
                            n1269 = case shown="True" w3700 {
                              tunnel: w3701 -> [_ w3705]
                              frame False {
                              }
                              frame True {
                                n1270 = local read "filename prefix"() -> (w3703:string)
                                n1271 = local read "data dir"() -> (w3704:path)
                                n1272 = call "preparebinaryfiles.vi"("filename prefix"=w3703, "data dir"=w3704, "timestamp"=w3705) -> ("full-filename"=w3702:string)  [unwired: 1 in]
                                n1273 = local write "full-filename"(w3702) -> ()
                              }
                            }
                          }
                          frame #3 {
                            n1274 = call "2pparameters.vi"("command"="get") -> ("params out"=w3707:T11)  [unwired: 1 in]
                            n1275 = Unbundle By Name(w3707) -> ("autoshutter"=w3708:bool)
                            n1276 = case shown="True" w3708 {
                              frame False {
                              }
                              frame True {
                                n1277 = call "shuttercontrol.vi"("command"="open") -> ()  [unwired: 1 in, 1 out]
                              }
                            }
                          }
                          frame #4 {
                            n1278 = flat-sequence {
                              frame #0 {
                                n1279 = call "runAI_img.vi"() -> ()  [unwired: 12 in]
                                n1280 = call "runCI.vi"() -> ()  [unwired: 12 in]
                                n1281 = call "runDO_img.vi"() -> ()  [unwired: 12 in]
                                n1282 = call "runAO_img.vi"() -> ()  [unwired: 12 in]
                              }
                              frame #1 {
                              }
                            }
                          }
                          frame #5 {
                            n1283 = while {
                              i -> [w3712]
                              stop <- w3710 stop-if-true
                              n1284 = local read "Stop"() -> (w3720:bool)
                              n1285 = local read "Exit"() -> (w3719:bool)
                              n1286 = Increment(x=w3712) -> (x+1=w3711:i32)
                              n1287 = local write "points recorded"(w3711) -> ()
                              n1288 = Or(x=w3720, y=w3719) -> (x .or. y?=w3718:bool)
                              n1289 = case shown="False" w3718 {
                                frame False {
                                n1290 = stacked-sequence {
                                frame #0 {
                                n1291 = call "collectCI_tt.vi"() -> ("size(s)"=w3727:i32)  [unwired: 3 in]
                                n1292 = local write "scol"(w3727) -> ()
                                n1293 = call "collectAI_tt_V2.vi"() -> ()  [unwired: 4 in]
                                }
                                frame #1 {
                                n1294 = local read "graph2list"() -> (w3732:u16)
                                n1295 = local read "graph1list"() -> (w3733:u16)
                                n1296 = To Unsigned Word Integer(number=w3732) -> (unsigned 16bit integer=w3735:u16)
                                n1297 = To Unsigned Word Integer(number=w3733) -> (unsigned 16bit integer=w3736:u16)
                                n1298 = local read "bin"() -> (w3740:dbl)
                                n1299 = call "dattotrace.vi"("graph2list"=w3735, "Current Average"=sgl 1.0, "graph1list"=w3736) -> ("trace2array out"=w3738:sgl[], "trace1array out"=w3737:sgl[])
                                n1300 = Array Size(array=w3738) -> (size(s)=w3741:i32)
                                n1301 = Divide(x=w3741, y=2) -> (x/y=w3743:dbl)
                                n1302 = Round To Nearest(number=w3743) -> (nearest integer value=w3745:dbl)
                                n1303 = script code="data=reshape(datain,[bin length(datain)./bin]);\ndataout=mean(data,1);"("bin"=w3740, "datain"=w3737) -> ("dataout"=w3739:dbl[])  [unwired: 1 in, 1 out]
                                n1304 = Array Size(array=w3739) -> (size(s)=w3750:i32)
                                n1305 = Delete From Array(array=w3738, length=w3745, index=0) -> (deleted portion=w3729:sgl[], array with subset deleted=w3728:sgl[])
                                n1306 = Divide(x=w3750, y=2) -> (x/y=w3748:dbl)
                                n1307 = Round To Nearest(number=w3748) -> (nearest integer value=w3746:dbl)
                                n1308 = Delete From Array(array=w3739, length=w3746, index=0) -> (deleted portion=w3730:dbl[], array with subset deleted=w3731:dbl[])
                                n1309 = local write "graph4"(w3728) -> ()
                                n1310 = local write "graph2"(w3731) -> ()
                                n1311 = local write "graph3"(w3729) -> ()
                                n1312 = local write "graph1"(w3730) -> ()
                                }
                                frame #2 {
                                n1313 = local read "save\ndata"() -> (w3751:bool)
                                n1314 = case shown="True" w3751 {
                                frame False {
                                }
                                frame True {
                                n1315 = call "savebinaryfiles.vi"() -> ()  [unwired: 1 in]
                                }
                                }
                                }
                                }
                                }
                                frame True {
                                }
                              }
                              n1316 = local read "continuous"() -> (w3715:bool)
                              n1317 = case shown="False" w3715 {
                                tunnel: w3711 -> [w3725 _]
                                tunnel: [w3724 FALSE] -> w3713
                                frame False {
                                n1318 = call "2pparameters.vi"("command"="get") -> ("params out"=w3722:T11)  [unwired: 1 in]
                                n1319 = Unbundle By Name(w3722) -> ("tt_cycles"=w3721:i32)
                                n1320 = Greater Or Equal?(x=w3725, y=w3721) -> (x >= y?=w3724:bool)
                                }
                                frame True {
                                }
                              }
                              n1321 = local read "Stop"() -> (w3717:bool)
                              n1322 = local read "Exit"() -> (w3716:bool)
                              n1323 = Or(x=w3717, y=w3716) -> (x .or. y?=w3714:bool)
                              n1324 = Or(x=w3714, y=w3713) -> (x .or. y?=w3710:bool)
                            }
                          }
                          frame #6 {
                            n1325 = call "stoperaseCI.vi"() -> ()  [unwired: 12 in]
                            n1326 = call "stoperaseDO_img.vi"() -> ()  [unwired: 12 in]
                            n1327 = call "stoperaseAO_img.vi"() -> ()  [unwired: 12 in]
                            n1328 = call "stoperaseAI_img.vi"() -> ()  [unwired: 12 in]
                          }
                          frame #7 {
                            w3754 = T22 2 items=["no dialog", "OK message", "continue or stop message", "OK message + warnings", "continue/stop + warnings"] ("type of dialog (OK msg:1)")
                            n1329 = call "displayerrors.vi"() -> ("error IO"=w3755:errorcluster)
                            n1330 = call <vilib>:"General Error Handler.vi"("type of dialog (OK msg:1)"=w3754, "error in (no error)"=w3755) -> ("error out"=w3753:errorcluster)  [unwired: 9 in, 4 out]
                            n1331 = call <vilib>:"Clear Errors.vi"("error in (no error)"=w3753) -> ("error out"=w3752:errorcluster)  [unwired: 5 in, 1 out]
                            n1332 = call "seterrors.vi"("error IO"=w3752) -> ()
                          }
                          frame #8 {
                            w3765 = FALSE ("Value (Signaling)")
                            n1333 = local read "save\ndata"() -> (w3760:bool)
                            n1334 = call "2pparameters.vi"("command"="get") -> ("params out"=w3758:T11)  [unwired: 1 in]
                            n1335 = Unbundle By Name(w3758) -> ("auto OD"=w3756:bool)
                            n1336 = case shown="True" w3760 {
                              tunnel: w3759 -> [_ w3772]
                              frame False {
                              }
                              frame True {
                                n1337 = local read "filename prefix"() -> (w3773:string)
                                n1338 = call "closebinaryfiles.vi"() -> ()  [unwired: 12 in]
                                n1339 = local read "data dir"() -> (w3774:path)
                                n1340 = call "saveparams.vi"("timestamp"=w3772, "filename prefix in"=w3773, "data dir in"=w3774) -> ()  [unwired: 1 in]
                              }
                            }
                            n1341 = case shown="True" w3756 {
                              frame False {
                              }
                              frame True {
                                n1342 = call "configuration.vi"("command"="get") -> ("config out"=w3768:T12)  [unwired: 2 in, 1 out]
                                n1343 = call "2pparameters.vi"("command"="get") -> ("params out"=w3771:T11)  [unwired: 1 in]
                                n1344 = Unbundle By Name(w3768) -> ("point OD"=w3766:u16)
                                n1345 = Unbundle By Name(w3771) -> ("ODfilt"=w3767:u16)
                                n1346 = call "filterwheelcontrol_nothorlabslib.vi"("Current OD filt"=w3766, "New ODfilt"=w3767) -> ()  [unwired: 1 in]
                              }
                            }
